vi "GetAlazar_SaveToFile_25 - ATS-SDK.vi"(1 "Digitizer Settings":T8={"Digitizer delay (us) "=0.0, "rf points per line"=2048, "lines per plane"=128, "Samp Rate (Hz)"=100000000.0, "Additional dig delay (us)"=0.0, "Voltage Scale"=0.4, "Pre-Looks"=0, "Offset delay (us)"=0.0, "bits A/D"=8, "Avg Num"=1, "DigTimeOut"=5.0, "Rel Dig Delay"=0.0, "Dig Ch"=0, "LeCroyCluster"={"LeCroy Channels"=[TRUE, FALSE, FALSE, FALSE], "LC read pt offset"=0.0, "Sweep Avg"=FALSE}, "Main Digitizer"=enum."NI Digitizer", "Dig Config"=enum."Single channel", "Digitizer ID Cluster"={"Acqiris/Alazar/SP ID"=[], "NI Instr Handles"=[], "LeCroy VISA"="", "GaGe Handle"={"Handle"=0, "Sample size"=0, "Resolution"=0, "Offset"=0, "Channels"=0, "Boards"=0}, "ATS Ref"="ATS9350", "Acqiris Address"=["PCI::INSTR0"], "ADQRef"=refnum, "adq_cu_ptr"=refnum}, "Trigger Settings"={"Trig Source"=1, "Trig Coupling"=0, "Trig Slope"=0, "Level (mV)"=1500.0}, "Bulk Acq"=FALSE, "Bulk Start Indexes"=[], "Data Ref RF"=refnum, "NI ID/Channel"=[], "Total Dig CH"=1, "Xtra Ann Trig delay (us)"=10.0, "Fix Z Delay?"=FALSE, "One Way Transmission?"=FALSE, "Data Ref Log"=refnum} {"Trigger Settings"."Trig Slope" items=["Positive", "Negative"]; "Trigger Settings"."Level (mV)" format="%.2f"; "Trigger Settings"."Trig Coupling" items=["DC 1 MOhm", "AC 1 MOhm", "DC 50 Ohm", "AC 50 Ohm"]; "Trigger Settings"."Trig Source" items=["Chan 1", "External"]; "Rel Dig Delay" format="%.2f"; "DigTimeOut" format="%.2f"; "Avg Num" min=1; "Offset delay (us)" format="%.2f"; "Additional dig delay (us)" format="%.2f"; "Digitizer delay (us)" format="%.2f"}, 3 "AlazarCluster":T12, 4 "Ann Array Params":T1={"Synth Foc?"=FALSE, "Focal Zones"=41, "Switch T/R"=0, "Trans Geometry (mm)"={"Transducer"=0, "Geo Focus"=12.0, "a (radius)"=3.0, "# of rings"=5, "kerf space "=0.1, "Center Freq"=12.0}, "Sub Ap Excite?"=FALSE, "Full Array Scan?"=FALSE, "Xmt/Rcv"={"XMIT"=[TRUE, TRUE, TRUE, TRUE, TRUE], "RCV"=[TRUE, TRUE, TRUE, TRUE, TRUE]}, "PulseSpacing (us)"=0.0, "Xmit Ring"=0, "XMIT CHS"=0, "RCV CHS"=0, "GPU?"=FALSE, "Save TIFF?"=FALSE, "downfactor"=1, "RCV 1CH"=0} {"RCV 1CH" items=["All", "1", "2", "3", "4", "5"]; "Trans Geometry (mm)"."Transducer" items=["6D 12R 40 MHz"=0, "10D 31R 20 MHz"=1, "10D 23R 20 MHz"=2, "6D 23R 40 MHz"=3, "4.5D 10.7R 40 MHz"=4, "9D 23.5R 20 MHz"=5, "9D 25.8R 20MHz"=6, "Enter"=99]; "Switch T/R" min=1 max=5 step=1}, 5 "errorin":errorcluster, 6 "File Array":string[](array[string]), 7 "Motion Settings":T4={"No Motion?"=FALSE, "Motion System"=enum."NI 735x", "Motion Bd ID"=1, "Motion Profile"="SMAC1", "# Axis"=1, "Reverse Z axis?"=TRUE, "SMAC Axis"=0, "scan pair"=enum."y-(x) scan", "RT fps"=6.0, "Steps per mm"=[1000, 1000, 1000, 1000], "Motor Parameters"={"velocity ct/s"=[10000.0, 10000.0, 10000.0, 50000.0], "accel ct/s^2"=[50000.0, 50000.0, 50000.0, 200000.0]}, "One Way Scan"=FALSE, "Reverse One Way Scan"=FALSE, "Global Position (mm)"=[], "Plane"=0, "Distance between\nscan lines (um)"=0.0, "Distance between\nscan planes (um)"=0.0, "number of scan planes"=1, "Total steps in line"=0, "Xtra plane\ndistance  (um)"=100, "Xtra planes "=1, "Add Axis"=FALSE, "overshoot cts"=200, "BKPT Shift"=0, "Scan Start Time (ms)"=0, "ESP VISA"="GPIB::1::INSTR", "3rd Axis"=1, "GL Ref Out"=refnum, "Galil Address"=""} {"3rd Axis" items=["x", "y", "z", "w"]; "Xtra planes" min=1; "Xtra plane\ndistance  (um)" min=0; "Distance between\nscan planes (um)" format="%.2f"; "Distance between\nscan lines (um)" format="%.2f"; "SMAC Axis" items=["None"=0, "Axis 1"=1, "Axis 2"=2, "Axis 3"=3, "Axis 4"=4, "Axis 5"=5, "Axis 6"=6, "Axis 7"=7, "Axis 8"=8, "Vector Space 1"=17, "Vector Space 2"=18, "Vector Space 3"=19, "Vector Space 4"=20]; "Motion Bd ID" min=1 max=32 step=1}, 8 "lines per plane":i32, 11 "Reverse?":bool) -> (12 "Gain Array":T13(array[cluster]), 13 "Raw VGain (scale)":dbl, 15 "VGain (dB)":dbl, 19 "error out":errorcluster)   [LabVIEW 2022 SP3]
uses:
  -DigitizerRoutines/DigitizerSettings.ctl
  -DigitizerRoutines/Digitizer.ctl
  -DigitizerRoutines/DigConfig.ctl
  -DigitizerRoutines/DigitizerID.ctl
  C:/Windows/System32/ADQAPI_dotNet_helper.dll
  Motion Controllers/NI_controller/-NI_MotionRoutines/MotionParameters.ctl
  Motion Controllers/NI_controller/-NI_MotionRoutines/MotionSys.ctl
  Motion Controllers/-MotionRoutines/ScanAxis.ctl
  Motion Controllers/-MotionRoutines/3rdAxis.ctl
  Annular Array/-AnnularRoutines/AnnularArray.ctl
  Annular Array/-AnnularRoutines/TransGeometry.ctl
  Annular Array/-AnnularRoutines/ArrayGeometry.ctl
  Motion Controllers/-MotionRoutines/MotionGlobals.vi
  -ScanSystem/DataHandling/ReverseData.vi
panel:
  out "read time":u32
  out "save time":u32
  out "Numeric":i32
  # "1-D and 2-D B scan settings"
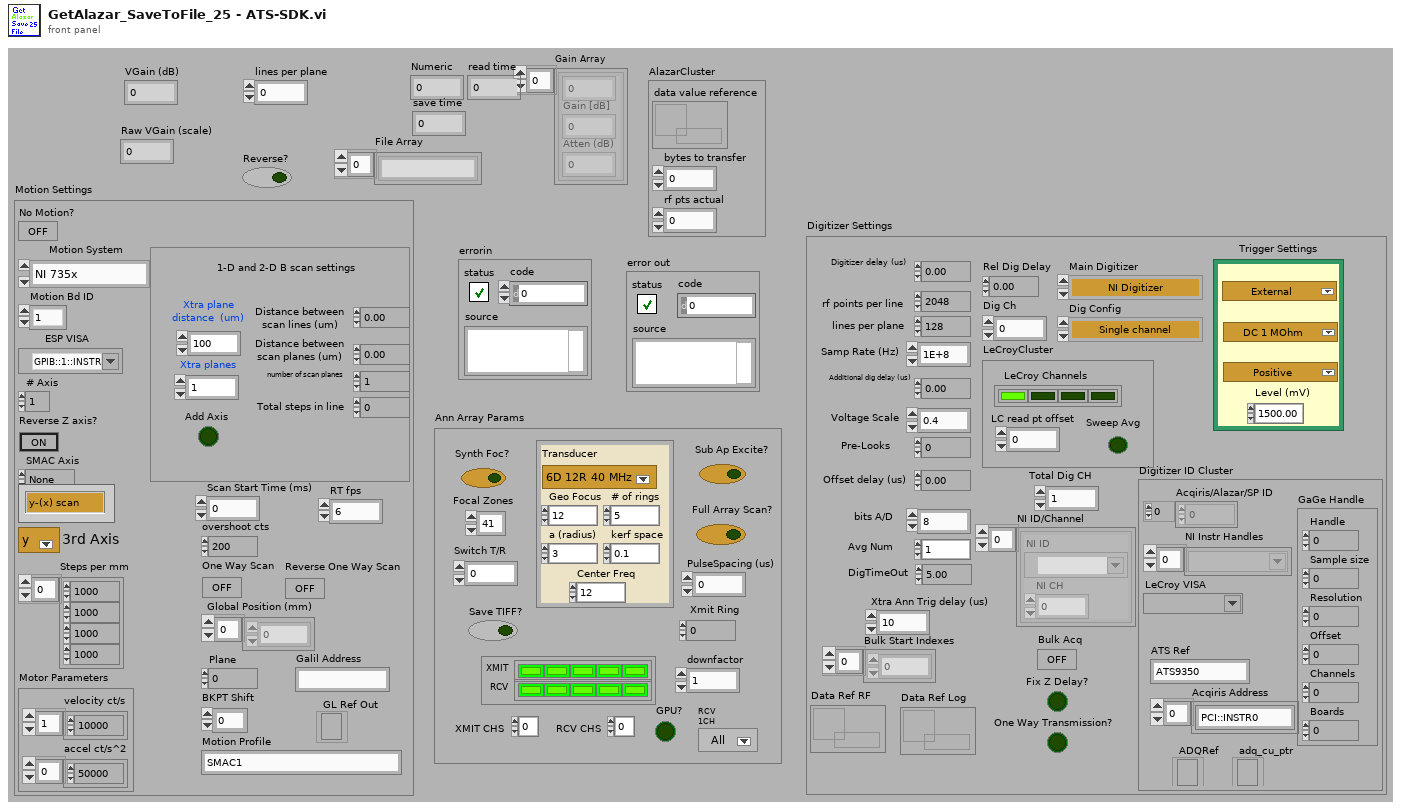
[diagram p1: front panel]
types:
  T1 = typedef "AnnularArray.ctl" = cluster{"Synth Foc?":bool, "Focal Zones":i16, "Switch T/R":i16, "Trans Geometry (mm)":T2, "Sub Ap Excite?":bool, "Full Array Scan?":bool, "Xmt/Rcv":cluster{"XMIT":bool[], "RCV":bool[]}, "PulseSpacing (us)":sgl, "Xmit Ring":i32, "XMIT CHS":u8, "RCV CHS":u8, "GPU?":bool, "Save TIFF?":bool, "downfactor":i32, "RCV 1CH":u16}
  T2 = typedef "TransGeometry.ctl" = cluster{"Transducer":T3, "Geo Focus":dbl, "a (radius)":dbl, "# of rings":i32, "kerf space ":dbl, "Center Freq":dbl}
  T3 = typedef "ArrayGeometry.ctl" = u16
  T4 = typedef "MotionParameters.ctl" = cluster{"No Motion?":bool, "Motion System":T5, "Motion Bd ID":u8, "Motion Profile":string, "# Axis":i8, "Reverse Z axis?":bool, "SMAC Axis":u16, "scan pair":T6, "RT fps":sgl, "Steps per mm":i32[], "Motor Parameters":cluster{"velocity ct/s":dbl[], "accel ct/s^2":dbl[]}, "One Way Scan":bool, "Reverse One Way Scan":bool, "Global Position (mm)":dbl[], "Plane":i32, "Distance between\nscan lines (um)":sgl, "Distance between\nscan planes (um)":sgl, "number of scan planes":i32, "Total steps in line":i32, "Xtra plane\ndistance  (um)":i32, "Xtra planes ":i32, "Add Axis":bool, "overshoot cts":i32, "BKPT Shift":i32, "Scan Start Time (ms)":u32, "ESP VISA":refnum<visa-resource-name>, "3rd Axis":T7, "GL Ref Out":refnum<k7>, "Galil Address":string}
  T5 = typedef "MotionSys.ctl" = enum16{"MM3000", "NI 735x", "Newport ESP", "No Motion Card", "Galil"}
  T6 = typedef "ScanAxis.ctl" = enum16{"y-(x) scan", "x-(y) scan", "z-(x) scan", "z-(y) scan", "y-(z) scan", "x-(z) scan", "w-(x) scan", "w-(y) scan", "w-(z) scan", "x-(w) scan", "y-(w) scan", "z-(w) scan"}
  T7 = typedef "3rdAxis.ctl" = u16
  T8 = typedef "DigitizerSettings.ctl" = cluster{"Digitizer delay (us) ":dbl, "rf points per line":i32, "lines per plane":i32, "Samp Rate (Hz)":dbl, "Additional dig delay (us)":dbl, "Voltage Scale":dbl, "Pre-Looks":i32, "Offset delay (us)":dbl, "bits A/D":i8, "Avg Num":i32, "DigTimeOut":sgl, "Rel Dig Delay":sgl, "Dig Ch":i32, "LeCroyCluster":cluster{"LeCroy Channels":bool[], "LC read pt offset":dbl, "Sweep Avg":bool}, "Main Digitizer":T9, "Dig Config":T10, "Digitizer ID Cluster":T11, "Trigger Settings":cluster{"Trig Source":u16, "Trig Coupling":u16, "Trig Slope":u16, "Level (mV)":dbl}, "Bulk Acq":bool, "Bulk Start Indexes":i32[], "Data Ref RF":refnum<data-value>, "NI ID/Channel":cluster{"NI ID":refnum<k15>, "NI CH":i32}[], "Total Dig CH":i32, "Xtra Ann Trig delay (us)":dbl, "Fix Z Delay?":bool, "One Way Transmission?":bool, "Data Ref Log":refnum<data-value>}
  T9 = typedef "Digitizer.ctl" = enum16{"Acqiris Digitizer", "NI Digitizer", "LeCroy", "GaGe", "AlazarTech", "No Digitizer", "Teledyne"}
  T10 = typedef "DigConfig.ctl" = enum16{"Single channel", "2 Chans w/ 2 Acqiris", "2 Chans w/ 1 Acqiris", "5-CH Pulser New", "5-CH pulser w/ ann array", "5-pass style ann array", "Empty"}
  T11 = typedef "DigitizerID.ctl" = cluster{"Acqiris/Alazar/SP ID":u32[], "NI Instr Handles":refnum<k15>[], "LeCroy VISA":refnum<visa-resource-name>, "GaGe Handle":cluster{"Handle":u32, "Sample size":u32, "Resolution":i32, "Offset":i32, "Channels":u32, "Boards":u32}, "ATS Ref":string, "Acqiris Address":string[], "ADQRef":refnum<k24>, "adq_cu_ptr":refnum<k24>}
  T12 = cluster{"data value reference":refnum<data-value>, "bytes to transfer":u32, "rf pts actual":u32}
  T13 = cluster{sgl, "Gain [dB]  ":sgl, "Atten (dB)":sgl}[]
  T14 = cluster{"wfm":i16[][], "max queue size (-1, unlimited)":i32}
  T15 = cluster{sgl, "Gain [dB]  ":sgl, "Atten (dB)":sgl}
  T16 = enum16{"open", "replace", "create", "open or create", "replace or create", "replace or create with confirmation"}
  T17 = enum16{"big-endian, network order", "native, host order", "little-endian"}
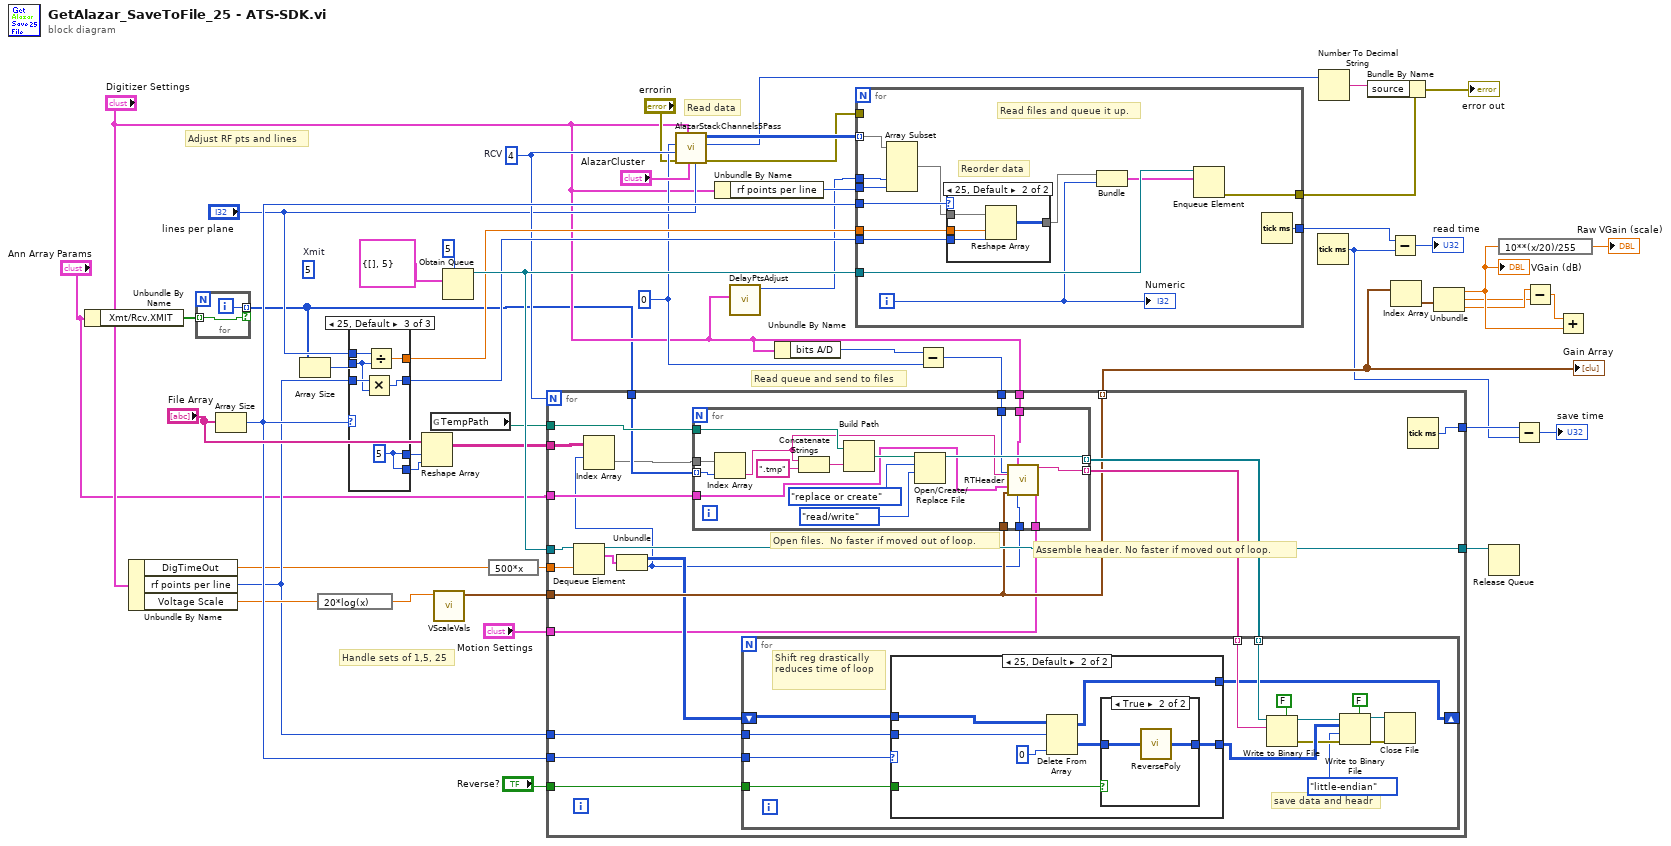
[diagram p0: block diagram]
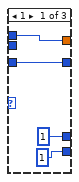
[diagram p3: hidden frame]
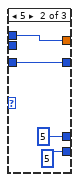
[diagram p4: hidden frame]
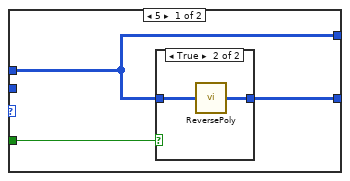
[diagram p5: hidden frame]
diagram:
  w11 = u16 0 ("Extra Shift")
  (unwired) 5  # Xmit
  w15 = 4  # RCV
  # "Read data"
  # "Adjust RF pts and lines"
  # "Handle sets of 1,5, 25"
  # "Read queue and send to files"
  n1 = Unbundle By Name("Ann Array Params") -> ("Xmt/Rcv.XMIT"=w3:bool[])
  n2 = Unbundle By Name("Digitizer Settings") -> ("DigTimeOut"=w17:sgl, "rf points per line"=w19:i32, "Voltage Scale"=w20:dbl)
  n3 = for {
    tunnel: w3 -> [w53] mode=indexing
    tunnel: [w54] -> w1 mode=indexing if=w53
    i -> [w54]
  }
  n4 = Array Size(array="File Array") -> (size(s)=w29:i32)
  n5 = Array Size(array=w1) -> (size(s)=w2:i32)
  n6 = expression code="20*log(x)"(w20) -> (w26:dbl)
  n7 = case shown="25, Default" w29 {
    tunnel: [1 5 w68] -> w34
    tunnel: [w57 w61 w64] -> w31
    tunnel: w19 -> [w57 w61 w65]
    tunnel: [w56 w60 w66] -> w32
    tunnel: "lines per plane" -> [w56 w60 w67]
    tunnel: [1 5 w68] -> w33
    tunnel: w2 -> [_ _ w63]
    frame 1 {
    }
    frame 5 {
    }
    frame 25, Default {
      w68 = 5
      n8 = Multiply(x=w65, y=w63) -> (x*y=w64:i32)
      n9 = Divide(x=w67, y=w63) -> (x/y=w66:dbl)
    }
  }
  n10 = Reshape Array("File Array", w34, w33) -> (w28:string[][])
  n11 = global read "MotionGlobals.vi" "TempPath"() -> (w27:path)
  n12 = call "VScaleVals.vi"("Full Scale"=w26) -> ("Voltage Scale"=w25:T15)  [unwired: 8 in, 2 out]
  n13 = Obtain Queue(max queue size (-1, unlimited)=5, element data type=T14 {"wfm"=[], "max queue size (-1, unlimited)"=5}) -> (queue out=w44:refnum<queue>)  [unwired: 3 in, 2 out]
  n14 = expression code="500*x"(w17) -> (w30:sgl)
  n15 = call "AlazarStackChannels5Pass.vi"("lines per plane"="lines per plane", "AlazarCluster"="AlazarCluster", "Digitizer Settings"="Digitizer Settings", "error in"="errorin", "Channels"=w15, "Extra Shift"=w11) -> ("error out"=w9:errorcluster, "Return Code"=w8:u32, "ChStackDataOut"=w13:i16[][][])  [unwired: 2 in, 1 out]
  n16 = Unbundle By Name("Digitizer Settings") -> ("rf points per line"=w7:i32)
  n17 = call "DelayPtsAdjust.vi"("Digitizer Settings"="Digitizer Settings") -> ("PostDelayCorrection"=w5:u32)  [unwired: 9 in, 1 out]
  n18 = Unbundle By Name("Digitizer Settings") -> ("bits A/D"=w18:i8)
  n19 = for {
    tunnel: w44 -> [w81]
    tunnel: [w79] -> w42
    tunnel: [w78] -> w24
    tunnel: w29 -> [w77]
    tunnel: w32 -> [w76]
    tunnel: w31 -> [w75]
    tunnel: w13 -> [w73] mode=indexing
    tunnel: w7 -> [w72]
    tunnel: w9 -> [_]
    tunnel: w5 -> [w69]
    i -> [w70]
    # "Read files and queue it up."
    # "Reorder data"
    n20 = Array Subset(array=w73, index (col)=w69, length (col)=w72) -> (w71:i16[][])  [unwired: 2 in]
    n21 = case shown="25, Default" w77 {
      tunnel: w75 -> [_ w86]
      tunnel: w71 -> [w82 w85]
      tunnel: [w82 w84] -> w74
      tunnel: w76 -> [_ w83]
      frame 0 {
      }
      frame 25, Default {
        n22 = Reshape Array(w85, w83, w86) -> (w84:i16[][])
      }
    }
    n23 = Bundle(w74, w70) -> (w80:cluster{i16[][], i32})  [unwired: 1 in]
    n24 = Enqueue Element(queue=w81, element=w80) -> (error out=w78:errorcluster)  [unwired: 2 in, 2 out]
    n25 = Tick Count (ms)() -> (millisecond timer value=w79:u32)
    "Numeric" <- w70
  }
  n26 = Subtract(x=w18, y=w11) -> (x-y=w21:u16)
  n27 = for {
    N: w15 -> [_]
    tunnel: w19 -> [w107]
    tunnel: "Reverse?" -> [w102]
    tunnel: [w94] -> w45 mode=indexing
    tunnel: w44 -> [w106]
    tunnel: [w104] -> w36
    tunnel: [w103] -> w41
    tunnel: w29 -> [w101]
    tunnel: w30 -> [w100]
    tunnel: w28 -> [w95]
    tunnel: w27 -> [w98]
    tunnel: w21 -> [w97]
    tunnel: w25 -> [w94]
    tunnel: "Digitizer Settings" -> [w92]
    tunnel: "Motion Settings" -> [w91]
    tunnel: "Ann Array Params" -> [w90]
    tunnel: w1 -> [w88]
    # "Open files.  No faster if moved out of loop."
    # "Assemble header. No faster if moved out of loop."
    n28 = Dequeue Element(queue=w106, timeout in ms (-1)=w100) -> (queue out=w104:refnum<queue>, element=w105:T14)  [unwired: 1 in, 2 out]
    n29 = Unbundle(w105) -> ("wfm"=w93:i16[][], "max queue size (-1, unlimited)"=w89:i32)
    n30 = Index Array(array=w95, index (row)=w89) -> (element=w87:string[])  [unwired: 1 in]
    n31 = for {
      tunnel: w87 -> [w109]
      tunnel: [w119] -> w99 mode=indexing
      tunnel: w98 -> [w118]
      tunnel: w94 -> [w117]
      tunnel: w97 -> [w116]
      tunnel: [w115] -> w96 mode=indexing
      tunnel: w92 -> [w114]
      tunnel: w91 -> [w113]
      tunnel: w89 -> [w112]
      tunnel: w90 -> [w111]
      tunnel: w88 -> [w110] mode=indexing
      n32 = Index Array(array=w109, index=w110) -> (element=w108:string)
      n33 = Concatenate Strings(w108, ".tmp") -> (w120:string)
      n34 = Build Path(base path=w118, name or relative path=w120) -> (appended path=w124:path)
      n35 = Open/Create/Replace File(file path (use dialog)=w124, operation (0:open)=T16."replace or create", access (0:read/write)=enum16{"read/write", "read-only", "write-only"}."read/write") -> (refnum out=w119:refnum<file>)  [unwired: 1 in, 4 out]
      n36 = call "RTHeader.vi"("Digitizer Settings"=w114, "Dig Word Size"=w116, "File Name In"=w108, "Ann Array Params"=w111, "Votage scaling"=w117, "Pulser Channel"=w112, "Motion Settings"=w113) -> ("Header String Out"=w115:string)  [unwired: 7 in, 1 out]
    }
    n37 = for {
      tunnel: w96 -> [w137] mode=indexing
      tunnel: w102 -> [w136]
      tunnel: w99 -> [w129] mode=indexing
      tunnel: w107 -> [w135]
      tunnel: w101 -> [w133]
      shift-right: [w126] -> _
      shift-left: w93 -> [w134]
      # "Shift reg drastically reduces time of loop"
      # "save data and headr"
      n38 = case shown="25, Default" w133 {
        tunnel: w136 -> [w142 w150]
        tunnel: [w141 w151] -> w132
        tunnel: w135 -> [_ w147]
        tunnel: w134 -> [w140 w149]
        tunnel: [w140 w148] -> w126
        frame 5 {
          n39 = case shown="True" w142 {
            tunnel: [w143 w145] -> w141
            tunnel: w140 -> [w143 w144]
            frame False {
            }
            frame True {
              n40 = call-poly "ReversePoly.vi"("Array in"=w144) -> ("Array out"=w145:i16[][])
            }
          }
        }
        frame 25, Default {
          n41 = Delete From Array(array=w149, length=w147, index (col)=0 ("index (row)")) -> (deleted portion=w152:i16[][], array with subset deleted=w148:i16[][])  [unwired: 1 in]
          n42 = case shown="True" w150 {
            tunnel: [w153 w155] -> w151
            tunnel: w152 -> [w153 w154]
            frame False {
            }
            frame True {
              n43 = call-poly "ReversePoly.vi"("Array in"=w154) -> ("Array out"=w155:i16[][])
            }
          }
        }
      }
      n44 = Write to Binary File(file (use dialog)=w129, data=w137, 5:FALSE ("prepend array or string size? (T)")) -> (refnum out=w128:refnum<file>, error out=w127:errorcluster)  [unwired: 3 in, 1 out]
      n45 = Write to Binary File(file (use dialog)=w128, data=w132, error in=w127, 5:FALSE ("prepend array or string size? (T)"), 9:T17."little-endian" ("byte order (0:big-endian, network order)")) -> (refnum out=w131:refnum<file>, error out=w130:errorcluster)  [unwired: 1 in, 1 out]
      n46 = Close File(refnum=w131, error in=w130) -> ()  [unwired: 2 out]
    }
    n47 = Tick Count (ms)() -> (millisecond timer value=w103:u32)
  }
  "Gain Array" <- w45
  n48 = Tick Count (ms)() -> (millisecond timer value=w40:u32)
  n49 = Number To Decimal String(number=w8) -> (decimal integer string=w23:string)  [unwired: 1 in]
  n50 = Bundle By Name(cluster=w24, "source"=w23) -> (→"error out":errorcluster)
  n51 = Subtract(x=w42, y=w40) -> (x-y=→"read time":u32)
  n52 = Index Array(array=w45) -> (element=w52:T15)  [unwired: 1 in]
  n53 = Unbundle(w52) -> (w51:sgl, "Gain [dB]"=w49:sgl, "Atten (dB)"=w50:sgl)
  "VGain (dB)" <- w51
  n54 = Release Queue(queue=w36) -> ()  [unwired: 2 in, 3 out]
  n55 = expression code="10**(x/20)/255"(w51) -> (→"Raw VGain (scale)":sgl)
  n56 = Subtract(x=w41, y=w40) -> (x-y=→"save time":u32)
  n57 = Subtract(x=w50, y=w49) -> (x-y=w48:sgl)
  n58 = Add(x=w48, y=w51) -> ()  [unwired: 1 out]
